vi "detector_get_data_dimensions.vi"(8 "error in (no error)":errorcluster, 11 "tt20 in":refnum<class "tt20.lvclass">) -> (0 "error out":errorcluster, 1 "data_type":T1, 2 "dims":u32[](array[numeric]), 3 "tt20 out":refnum<class "tt20.lvclass">)   [LabVIEW 2015, in "tt20.lvclass"]
uses:
  tt20.lvclass
  detector/data_types_tdef.ctl
  tt20.lvclass/tt20.ctl
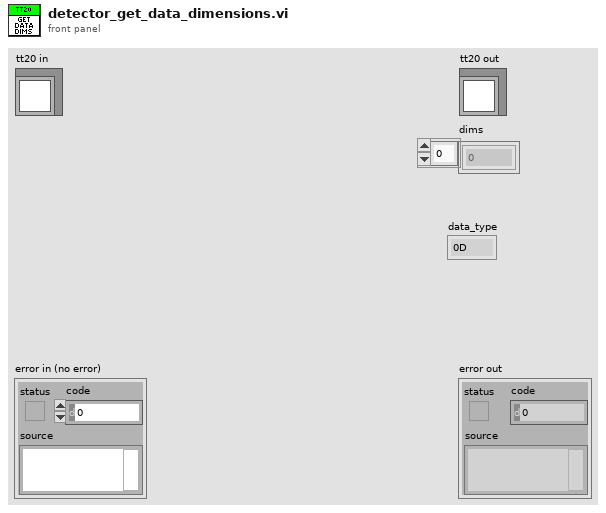
[diagram p1: front panel]
types:
  T1 = typedef "data_types_tdef.ctl" = enum16{"0D", "1D", "2D"}
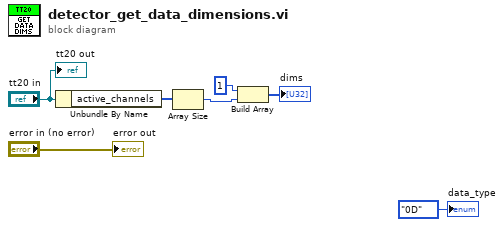
[diagram p0: block diagram]
diagram:
  n1 = Unbundle By Name("tt20 in") -> ("active_channels"=w7:u32[])
  n2 = Array Size(array=w7) -> (size(s)=w2:i32)
  n3 = Build Array(u32 1 ("element"), w2) -> (→"dims":u32[])
  "error out" <- "error in (no error)"
  "tt20 out" <- "tt20 in"
  "data_type" <- data_types_tdef."0D" ("data_type")
